vi "Format Knock Cylinders into Table.vi"(11 "Knock Cylinders":T1[](array[typedef])) -> (3 "Table":string[][](array[string]))   [LabVIEW 2017, in "Engine Simulation Toolkit System Explorer.lvlib"]
uses:
  Engine Simulation Toolkit System Explorer.lvlib
  Knock Cylinder.ctl
  Shared/Constants and GUIDs.vi
  Shared/Engine Simulation Toolkit Shared.lvlib
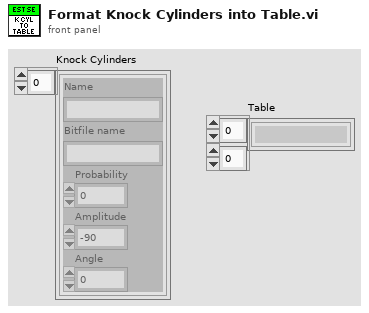
[diagram p1: front panel]
types:
  T1 = typedef "Engine Simulation Toolkit System Explorer.lvlib/Knock Cylinder.ctl" = cluster{"Name":string, "Bitfile name":string, "Probability":dbl, "Amplitude":dbl, "Angle":dbl}
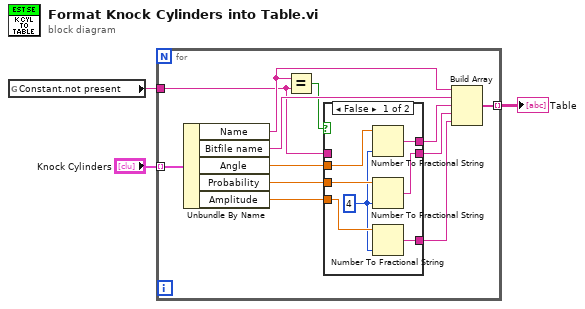
[diagram p0: block diagram]
diagram:
  n1 = global read "Constants and GUIDs.vi" "Constant.not present"() -> (w1:string)
  n2 = for {
    tunnel: "Knock Cylinders" -> [w15] mode=indexing
    tunnel: [w14] -> w2 mode=indexing
    tunnel: w1 -> [w8]
    n3 = Unbundle By Name(w15) -> ("Name"=w12:string, "Bitfile name"=w13:string, "Angle"=w5:dbl, "Probability"=w7:dbl, "Amplitude"=w9:dbl)
    n4 = Equal?(x=w12, y=w8) -> (x = y?=w11:bool)
    n5 = case shown="False" w11 {
      tunnel: [w20 w23] -> w10
      tunnel: w9 -> [w21 _]
      tunnel: w8 -> [_ w23]
      tunnel: w7 -> [w22 _]
      tunnel: [w19 w23] -> w6
      tunnel: w5 -> [w18 _]
      tunnel: [w16 w23] -> w4
      frame False {
        w17 = i16 4 ("precision (6)")
        n6 = Number To Fractional String(number=w18, precision (6)=w17) -> (F-format string=w16:string)  [unwired: 2 in]
        n7 = Number To Fractional String(number=w22, precision (6)=w17) -> (F-format string=w19:string)  [unwired: 2 in]
        n8 = Number To Fractional String(number=w21, precision (6)=w17) -> (F-format string=w20:string)  [unwired: 2 in]
      }
      frame True {
      }
    }
    n9 = Build Array(w12, w13, w4, w6, w10) -> (w14:string[])
  }
  "Table" <- w2
